vi "ATS_Inputs_4Ch.vi"(10 "Channels_Input":T1 {"Range" items=["20mV", "40mV", "50mV", "80mV", "100mV", "200mV", "400mV", "500mV", "800mV", "1 V", "1.25 V", "2 V", "4 V", "5 V", "8 V", "10 V", "16 V", "20 V", "40 V", "HiFi"]}, 11 "DeviceIn":i32) -> (0 "Return Code":u32, 1 "ChB_Range":dbl format="%.3f", 2 "ChA_Range":dbl format="%.3f", 3 "DeviceOut":i32, 4 "Channels_Range":dbl[](array[numeric]) format="%.3f")   [LabVIEW 2015]
doc: "_____AlazarTech, Scope_____\n\nConfigure the input channels.\n\n- Channel\n- Coupling\n- Range\n- Impedance"
uses:
  ATS_ctl/ATS_InputArray.ctl
  ATS_ctl/InputCtrl.ctl
  ATS_ctl/Coupling.ctl
  ATS_ctl/Range.ctl
  ATS_ctl/Impedance.ctl
  ATS_ctl/Bandwidth.ctl
  ATS_ctl/ATS_Global_Ctrl.ctl
  ATS_ctl/ATS_Channel.ctl
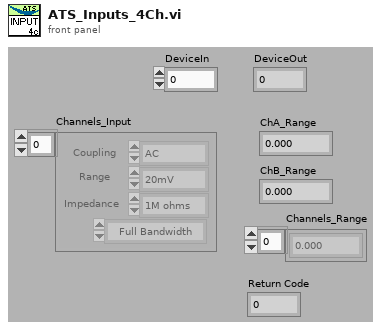
[diagram p1: front panel]
types:
  T1 = typedef "ATS_InputArray.ctl" = T2[]
  T2 = typedef "InputCtrl.ctl" = cluster{"Coupling":T3, "Range":T4, "Impedance":T5, "Bandwidth":T6}
  T3 = typedef "Coupling.ctl" = enum16{"AC", "DC"}
  T4 = typedef "Range.ctl" = u32
  T5 = typedef "Impedance.ctl" = enum16{"1M ohms", "50 ohms"}
  T6 = typedef "Bandwidth.ctl" = enum16{"Full Bandwidth", "Reduce Bandwidth"}
  T7 = typedef "ATS_Channel.ctl" = enum16{"Channel_A", "Channel_B", "Channel_C", "Channel_D"}
  T8 = typedef "ATS_Global_Ctrl.ctl" = enum16{"Init_Device", "Clear_ALL", "Set", "Get"}
  T9 = typedef "ATS_Set_Value.ctl" = cluster{"Clock (s)":dbl, "RangeA (v)":dbl, "RangeB (v)":dbl, "Ranges (v)":dbl[]}
  T10 = typedef "ATS_Global_4Ch.ctl" = cluster{"Record":T11, "Clock":T12, "Inputs":T1, "Trigger":T16}
  T11 = typedef "Record.ctl" = cluster{"Count":u32, "Presize":u32, "Length":u32}
  T12 = typedef "Clock.ctl" = cluster{"ClckSource":T13, "ClckRate":T14, "ClckEdge":T15, "Decimation":u32}
  T13 = typedef "ClockSource.ctl" = enum16{"Internal", "External", "Medium Ext.", "Slow Ext.", "Ext. AC", "Ext. DC", "Ext. (PLL)"}
  T14 = typedef "ClockRate.ctl" = u32
  T15 = typedef "ClockEdge.ctl" = u16
  T16 = typedef "ATS_Trigger_4Ch.ctl" = cluster{"TrigOperation":T17, "Timeout (s)":dbl, "Trig. Delay":u32, "Engine X":T18, "Engine Y":T18, "ExtTrigControl":T20}
  T17 = typedef "TriggerOperation.ctl" = enum16{"Only X", "Only Y", "X or Y", "X and Y", "X xor Y", "X and not Y", "not X and Y"}
  T18 = typedef "ATS_TriggerEngine_4Ch.ctl" = cluster{"Source":T19, "Slope":enum32{"Positive", "Negative"}, "Level":u32}
  T19 = typedef "ATS_TriggerSource_4Ch.ctl" = enum32{"Chan_A", "Chan_B", "External", "Disable", "Chan_C", "Chan_D"}
  T20 = typedef "ExtTrigger.ctl" = cluster{"Coupling":T3, "Range":T21}
  T21 = typedef "ExtTrigRange.ctl" = enum16{"1 V", "5 V", "TTL"}
  T22 = typedef "Device_Info.ctl" = cluster{"Handle":u32, "Board":string, "CPLD":string, "MemorySize":u32, "SampleSize":u8, "ID":i32, "High_Memory":bool, "Chan/Board":u8}
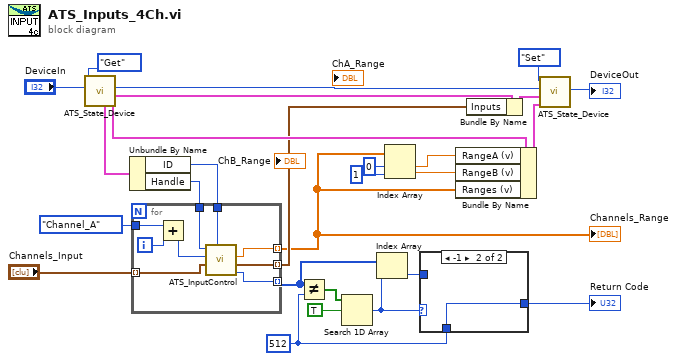
[diagram p0: block diagram]
diagram:
  w1 = u32 512 ("Return Code")
  n1 = call "ATS_State_Device.vi"("DeviceIn"="DeviceIn", "ATS_GBL_Ctrl"=ATS_Global_Ctrl."Get") -> ("Ref_Out"=w21:T9, "SetupOut"=w20:T10, "DeviceOut"=w24:i32, "DevInfo_Out"=w16:T22)  [unwired: 4 in, 2 out]
  n2 = Unbundle By Name(w16) -> ("ID"=w13:i32, "Handle"=w14:u32)
  n3 = for {
    tunnel: "Channels_Input" -> [w31] mode=indexing
    tunnel: ATS_Channel."Channel_A" ("Channel") -> [w34]
    tunnel: w14 -> [w33]
    tunnel: w13 -> [w32]
    tunnel: [w30] -> w12 mode=indexing
    tunnel: [w29] -> w9 mode=indexing
    tunnel: [w28] -> w4 mode=indexing
    i -> [w35]
    n4 = Add(x=w34, y=w35) -> (x+y=w36:i32)
    n5 = call "ATS_InputControl.vi"("ID"=w32, "InputControl"=w31, "Channel"=w36, "HandleIn"=w33) -> ("Return Code"=w28:u32, "OutputControl"=w30:T2, "Range_Value"=w29:dbl)  [unwired: 4 in, 1 out]
  }
  "Channels_Range" <- w9
  n6 = Not Equal?(x=w4, y=w1) -> (x != y?=w6:bool[])
  n7 = Search 1D Array(1D array=w6, element=TRUE) -> (index of element=w3:i32)  [unwired: 1 in]
  n8 = Index Array(array=w4, index=w3) -> (element=w2:u32)
  n9 = Index Array(array=w9, index #1=0 ("index"), index #2=1 ("index")) -> (element #1=w11:dbl, element #2=w10:dbl)
  n10 = case shown="-1" w3 {
    tunnel: [w37 w38] -> w19
    tunnel: w2 -> [w37 _]
    tunnel: w1 -> [_ w38]
    frame 0, Default {
    }
    frame -1 {
      # "no error on ChA"
    }
  }
  "Return Code" <- w19
  n11 = Bundle By Name(cluster=w21, "RangeA (v)"=w11, "RangeB (v)"=w10, "Ranges (v)"=w9) -> (w18:T9)
  n12 = Bundle By Name(cluster=w20, "Inputs"=w12) -> (w22:T10)
  n13 = call "ATS_State_Device.vi"("Ref_In"=w18, "SetupIn"=w22, "DeviceIn"=w24, "ATS_GBL_Ctrl"=ATS_Global_Ctrl."Set") -> ("DeviceOut"=→"DeviceOut":i32)  [unwired: 2 in, 5 out]
